vi "Read Collision Grid.vi"(8 "error in (no error)":errorcluster, 11 "PhysicsSystem in":refnum<class "PhysicsSystem.lvclass">) -> (0 "error out":errorcluster, 2 "Collision Grid out":refnum<class "CollisionGrid.lvclass">, 3 "PhysicsSystem out":refnum<class "PhysicsSystem.lvclass">)   [LabVIEW 2022 SP3, in "PhysicsSystem.lvclass"]
uses:
  PhysicsSystem.lvclass
  PhysicsSystem.lvclass/PhysicsSystem.ctl
  Objects/Collisions/CollisionGrid/CollisionGrid.lvclass
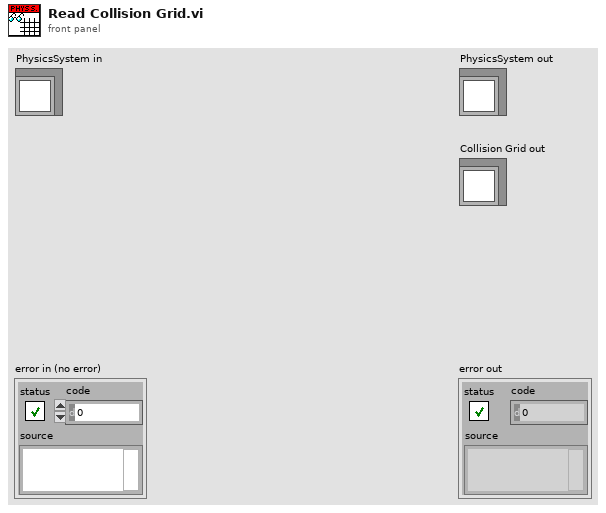
[diagram p1: front panel]
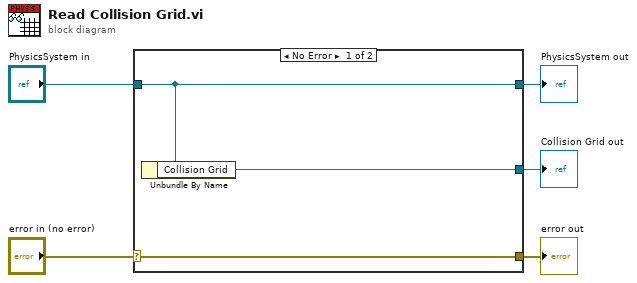
[diagram p0: block diagram]
diagram:
  n1 = case shown="No Error" "error in (no error)" {
    selector: "error in (no error)" -> [w8 w9]
    tunnel: [w8 w9] -> w4
    tunnel: [w7 w10] -> w2
    tunnel: "PhysicsSystem in" -> [w7 w10]
    tunnel: [w6 _] -> w1
    frame No Error {
      n2 = Unbundle By Name(w7) -> ("Collision Grid"=w6:refnum<class "CollisionGrid.lvclass">)
    }
    frame Error {
    }
  }
  "error out" <- w4
  "PhysicsSystem out" <- w2
  "Collision Grid out" <- w1
